vi "04.1 Creating Property Nodes.vi"() -> ()   [LabVIEW 2019]
panel:
  out "Tip Strip":string
  out "Visible":bool
  in  "Disable":T1(ring)
  in  "Numeric":dbl
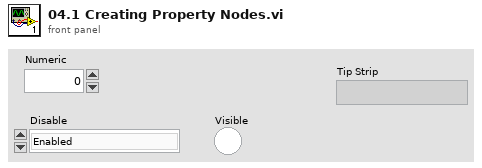
[diagram p1: front panel]
types:
  T1 = enum8{"Enabled", "Disabled", "Disabled and Grayed Out"}
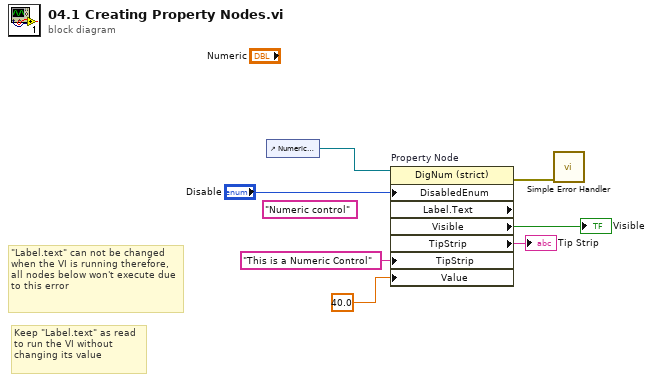
[diagram p0: block diagram]
diagram:
  (unwired) "Numeric control" ("Label.Text")
  # "Keep \"Label.text\" as read to run the VI without changing its value"
  # "\"Label.text\" can not be changed when the VI is running therefore, all nodes below won't execute due to this error"
  n1 = control-ref of="Numeric reference"() -> (w7:refnum<vi>)
  n2 = property on="Property Node" class="DigNum (strict)" props=["DisabledEnum", "Label", "Text", "Visible", "TipStrip", "TipStrip", "Value"](reference=w7, "DisabledEnum"="Disable", "TipStrip"="This is a Numeric Control" ("Tip Strip"), "Value"=40.0) -> (error out=w5:errorcluster, "Visible"=→"Visible":bool, "TipStrip"=→"Tip Strip":string)  [unwired: 1 in, 2 out]
  n3 = call <vilib>:"Simple Error Handler.vi"("error in (no error)"=w5) -> ()  [unwired: 4 in, 5 out]
